vi "Get SMO PGSQL Log Paths.vi"(5 "getAll Cluster":variant, 7 "Default Paths":string, 8 "error in (no error)":errorcluster, 11 "FP-TC-Shared in":refnum<class "FP-TC-Shared.lvclass">) -> (0 "error out":errorcluster, 2 "Paths":string, 3 "FP-TC-Shared out":refnum<class "FP-TC-Shared.lvclass">)   [LabVIEW 2019, in "FP-TC-Shared.lvclass"]
uses:
  FP-TC-Shared.lvclass
  typedefs/Default PGSQL Paths.ctl
  FP-TC-Shared.lvclass/FP-TC-Shared.ctl
  <userlib>/LevyLab/Configuration/Configuration.lvclass/Configuration.ctl
  73a01e10-25b7-4c77-987b-687e2f0d43b2.vi
  <vilib>/Utility/Data Type/Get Type Information.vi
  <vilib>/Utility/Data Type/Get Numeric Information.vi
  <userlib>/_OpenG.lib/lvdata/lvdata.llb/Unwrap VVariant__ogtk.vi
  <userlib>/LevyLab/Instrument Framework/Instrument Types/Cryostat/Instrument.Cryostat.lvclass
  <userlib>/LevyLab/Configuration/Configuration.lvclass
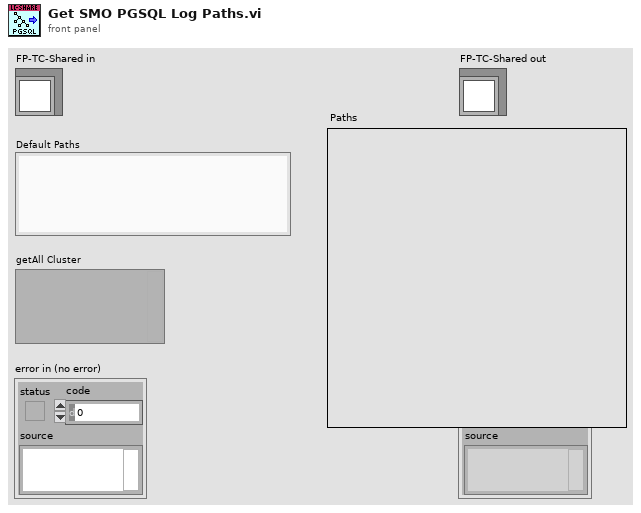
[diagram p1: front panel]
types:
  T1 = typedef "FP-TC-Shared.lvclass/Default PGSQL Paths.ctl" = cluster{"CF.TC":string, "CF.TC.Z":string, "CF.FP":string, "MNK.TC":string, "MNK.TC.Z":string, "MNK.FP":string}
  T2 = typedef "FP-TC-Shared.lvclass/LC Type--Enum.ctl" = enum16{"CF.TC", "CF.TC.Z", "CF.FP", "MNK.TC", "MNK.TC.Z", "MNK.FP"}
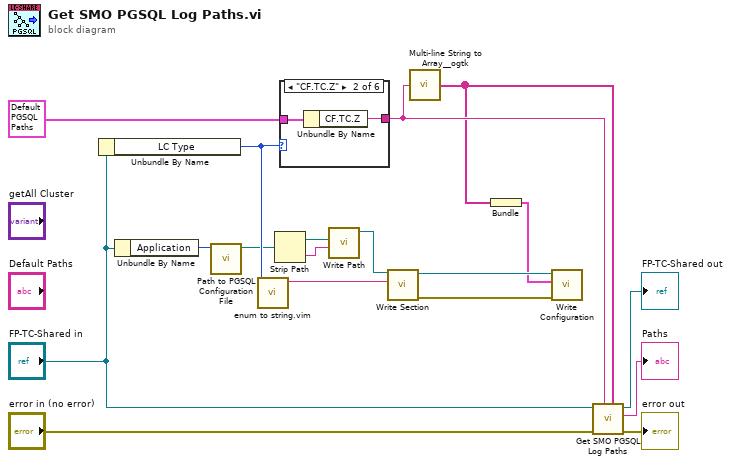
[diagram p0: block diagram]
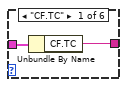
[diagram p2: hidden frame]
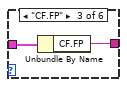
[diagram p3: hidden frame]
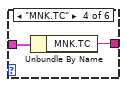
[diagram p4: hidden frame]
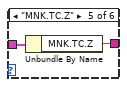
[diagram p5: hidden frame]
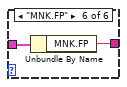
[diagram p6: hidden frame]
diagram:
  n1 = Unbundle By Name("FP-TC-Shared in") -> ("LC Type"=w12:T2)
  n2 = Unbundle By Name("FP-TC-Shared in") -> ("Application"=w6:enum16{"TC", "FP"})
  n3 = call "Path to PGSQL Configuration File.vi"("Application"=w6) -> ("appended path"=w2:path)  [unwired: 10 in]
  n4 = call "enum to string.vim"("enum in"=w12) -> ("string out"=w11:string)  [unwired: 9 in, 1 out]
  n5 = Strip Path(path=w2) -> (stripped path=w4:path, name=w5:string)
  n6 = case shown="\"CF.TC.Z\"" w12 {
    tunnel: T1 {"CF.TC"="llab_015:d001(Leiden CF900--CF_TC_R0(ohms))\nllab_015:d002(Leiden CF900--CF_TC_R1(ohms))\nllab_015:d003(Leiden CF900--CF_TC_R2(ohms))\nllab_015:d004(Leiden CF900--CF_TC_R3(ohms))\nllab_015:d005(Leiden CF900--CF_TC_R4(ohms))\nllab_015:d006(Leiden CF900--CF_TC_R5(ohms))\nllab_015:d007(Leiden CF900--CF_TC_R6(ohms))\nllab_015:d008(Leiden CF900--CF_TC_R7(ohms))\nllab_015:d009(Leiden CF900--CF_TC_T0(mK))\nllab_015:d010(Leiden CF900--CF_TC_T1(mK))\nllab_015:d011(Leiden CF900--CF_TC_T2(mK))\nllab_015:d012(Leiden CF900--CF_TC_T3(mK))\nllab_015:d013(Leiden CF900--CF_TC_T4(mK))\nllab_015:d014(Leiden CF900--CF_TC_T5(mK))\nllab_015:d015(Leiden CF900--CF_TC_T6(mK))\nllab_015:d016(Leiden CF900--CF_TC_T7(mK))\nllab_015:d017(Leiden CF900--CF_TC_I0(Amp))\nllab_015:d018(Leiden CF900--CF_TC_I1(Amp))\nllab_015:d019(Leiden CF900--CF_TC_I2(Amp))\nllab_015:d020(Leiden CF900--CF_TC_I3(Amp))\nllab_015:v000(Leiden CF900--CF_TC_description())\nllab_015:v001(Leiden CF900--CF_TC_calibration())", "CF.TC.Z"="llab_015:d021(Leiden CF900--CF_TC_Z_R0(ohms))\nllab_015:d022(Leiden CF900--CF_TC_Z_R1(ohms))\nllab_015:d023(Leiden CF900--CF_TC_Z_R2(ohms))\nllab_015:d024(Leiden CF900--CF_TC_Z_R3(ohms))\nllab_015:d025(Leiden CF900--CF_TC_Z_R4(ohms))\nllab_015:d026(Leiden CF900--CF_TC_Z_R5(ohms))\nllab_015:d027(Leiden CF900--CF_TC_Z_R6(ohms))\nllab_015:d028(Leiden CF900--CF_TC_Z_R7(ohms))\nllab_015:d029(Leiden CF900--CF_TC_Z_R8(ohms))\nllab_015:d030(Leiden CF900--CF_TC_Z_R9(ohms))\nllab_015:d031(Leiden CF900--CF_TC_Z_T0(mK))\nllab_015:d032(Leiden CF900--CF_TC_Z_T1(mK))\nllab_015:d033(Leiden CF900--CF_TC_Z_T2(mK))\nllab_015:d034(Leiden CF900--CF_TC_Z_T3(mK))\nllab_015:d035(Leiden CF900--CF_TC_Z_T4(mK))\nllab_015:d036(Leiden CF900--CF_TC_Z_T5(mK))\nllab_015:d037(Leiden CF900--CF_TC_Z_T6(mK))\nllab_015:d038(Leiden CF900--CF_TC_Z_T7(mK))\nllab_015:d039(Leiden CF900--CF_TC_Z_T8(mK))\nllab_015:d040(Leiden CF900--CF_TC_Z_T9(mK))\nllab_015:v002(Leiden CF900--CF_TC_Z_description())\nllab_015:v003(Leiden CF900--CF_TC_Z_calibration())", "CF.FP"="llab_011:d000(Leiden CF FP--CF_FP_P1(mbar))\nllab_011:d001(Leiden CF FP--CF_FP_P2(mbar))\nllab_011:d002(Leiden CF FP--CF_FP_P3(mbar))\nllab_011:d003(Leiden CF FP--CF_FP_P4(mbar))\nllab_011:d004(Leiden CF FP--CF_FP_P5(mbar))\nllab_011:d005(Leiden CF FP--CF_FP_P6(mbar))\nllab_011:d006(Leiden CF FP--CF_FP_P7(mbar))\nllab_011:d007(Leiden CF FP--CF_FP_Flow())\nllab_011:d008(Leiden CF FP--CF_FP_MG0(mbar))\nllab_011:d009(Leiden CF FP--CF_FP_MG1(mbar))\nllab_011:d010(Leiden CF FP--CF_FP_MG2(mbar))\nllab_011:d011(Leiden CF FP--CF_FP_MG3(mbar))\nllab_011:d012(Leiden CF FP--CF_FP_MG4(mbar))\nllab_011:d013(Leiden CF FP--CF_FP_MG5(mbar))\nllab_011:d014(Leiden CF FP--CF_FP_PT_on())\nllab_011:d015(Leiden CF FP--CF_FP_PT_W_in_T(K))\nllab_011:d016(Leiden CF FP--CF_FP_PT_W_out_T(K))\nllab_011:d017(Leiden CF FP--CF_FP_PT_He_T(K))\nllab_011:d018(Leiden CF FP--CF_FP_PT_oil_T(K))\nllab_011:d019(Leiden CF FP--CF_FP_PT_P_Low(bar))\nllab_011:d020(Leiden CF FP--CF_FP_PT_P_High(bar))\nllab_011:d021(Leiden CF FP--CF_FP_PT_current(A))\nllab_011:d022(Leiden CF FP--CF_FP_state0())\nllab_011:d023(Leiden CF FP--CF_FP_state1())\nllab_011:d024(Leiden CF FP--CF_FP_state2())\nllab_011:v000(Leiden CF FP--CF_FP_STATE())", "MNK.TC"="llab_024:d020(MNK_18T--MNK_TC_R0(ohms))\nllab_024:d039(MNK_18T--MNK_TC_R1(ohms))\nllab_024:d021(MNK_18T--MNK_TC_R2(ohms))\nllab_024:d022(MNK_18T--MNK_TC_R3(ohms))\nllab_024:d037(MNK_18T--MNK_TC_R4(ohms))\nllab_024:d023(MNK_18T--MNK_TC_R5(ohms))\nllab_024:d024(MNK_18T--MNK_TC_R6(ohms))\nllab_024:d025(MNK_18T--MNK_TC_R7(ohms))\nllab_024:d026(MNK_18T--MNK_TC_T0(mK))\nllab_024:d027(MNK_18T--MNK_TC_T1(mK))\nllab_024:d028(MNK_18T--MNK_TC_T2(mK))\nllab_024:d029(MNK_18T--MNK_TC_T3(mK))\nllab_024:d030(MNK_18T--MNK_TC_T4(mK))\nllab_024:d038(MNK_18T--MNK_TC_T5(mK))\nllab_024:d031(MNK_18T--MNK_TC_T6(mK))\nllab_024:d032(MNK_18T--MNK_TC_T7(mK))\nllab_024:d033(MNK_18T--MNK_TC_I0(Amp))\nllab_024:d034(MNK_18T--MNK_TC_I1(Amp))\nllab_024:d035(MNK_18T--MNK_TC_I2(Amp))\nllab_024:d036(MNK_18T--MNK_TC_I3(Amp))\nllab_024:v005(MNK_18T--MNK_TC_description())\nllab_024:v006(MNK_18T--MNK_TC_calibration())", "MNK.TC.Z"="llab_024:d040(MNK_18T--MNK_Cstill_Z(pF))\nllab_024:d041(MNK_18T--MNK_CMN-187_Z(H))\nllab_024:d042(MNK_18T--MNK_Cstill_T(mK))\nllab_024:d043(MNK_18T--MNK_CMN-187_T(mK))\nllab_024:v005(MNK_18T--MNK_TC_Z_description())\nllab_024:v006(MNK_18T--MNK_TC_Z_calibration())", "MNK.FP"="llab_016:d000(Leiden MNK Front Panel--MNK_FP_P1(mbar))\nllab_016:d001(Leiden MNK Front Panel--MNK_FP_P2(mbar))\nllab_016:d002(Leiden MNK Front Panel--MNK_FP_P3(mbar))\nllab_016:d003(Leiden MNK Front Panel--MNK_FP_P4(mbar))\nllab_016:d004(Leiden MNK Front Panel--MNK_FP_P5(mbar))\nllab_016:d005(Leiden MNK Front Panel--MNK_FP_P6(mbar))\nllab_016:d006(Leiden MNK Front Panel--MNK_FP_P7(mbar))\nllab_016:d013(Leiden MNK Front Panel--MNK_FP_Flow())\nllab_016:d007(Leiden MNK Front Panel--MNK_FP_MG0(mbar))\nllab_016:d008(Leiden MNK Front Panel--MNK_FP_MG1(mbar))\nllab_016:d009(Leiden MNK Front Panel--MNK_FP_MG2(mbar))\nllab_016:d010(Leiden MNK Front Panel--MNK_FP_MG3(mbar))\nllab_016:d011(Leiden MNK Front Panel--MNK_FP_MG4(mbar))\nllab_016:d012(Leiden MNK Front Panel--MNK_FP_MG5(mbar))\nllab_016:d014(Leiden MNK Front Panel--MNK_FP_state0())\nllab_016:d015(Leiden MNK Front Panel--MNK_FP_state1())\nllab_016:d016(Leiden MNK Front Panel--MNK_FP_state2())\nllab_016:v000(Leiden MNK Front Panel--MNK_FP_STATE())"} ("PGSQL Paths") -> [w20 w22 w24 w26 w28 w30]
    tunnel: [w19 w21 w23 w25 w27 w29] -> w13
    frame "CF.TC" {
      n7 = Unbundle By Name(w20) -> ("CF.TC"=w19:string)
    }
    frame "CF.TC.Z" {
      n8 = Unbundle By Name(w22) -> ("CF.TC.Z"=w21:string)
    }
    frame "CF.FP" {
      n9 = Unbundle By Name(w24) -> ("CF.FP"=w23:string)
    }
    frame "MNK.TC" {
      n10 = Unbundle By Name(w26) -> ("MNK.TC"=w25:string)
    }
    frame "MNK.TC.Z" {
      n11 = Unbundle By Name(w28) -> ("MNK.TC.Z"=w27:string)
    }
    frame "MNK.FP" {
      n12 = Unbundle By Name(w30) -> ("MNK.FP"=w29:string)
    }
  }
  n13 = call <userlib>:"Write Path.vi"("Filename [Configuration.ini]"=w5, "Path"=w4) -> ("Configuration out"=w1:refnum<class "Configuration.lvclass">)  [unwired: 8 in, 1 out]
  n14 = call <userlib>:"Write Section.vi"("Section"=w11, "Configuration in"=w1) -> ("error out"=w10:errorcluster, "Configuration out"=w9:refnum<class "Configuration.lvclass">)  [unwired: 8 in]
  n15 = call <userlib>:"Multi-line String to Array__ogtk.vi"("string"=w13) -> ("lines"=w8:string[])
  n16 = Bundle("lines"=w8) -> (w7:cluster{"lines":string[]})  [unwired: 1 in]
  n17 = call <userlib>:"Write Configuration.vi"("error in (no error)"=w10, "Variant"=w7, "Configuration in"=w9) -> ()  [unwired: 7 in, 2 out]
  n18 = call-parent "Get SMO PGSQL Log Paths.vi"("getAll Cluster"=w8, "Default Paths"=w13, "error in (no error)"="error in (no error)", "Instrument in"="FP-TC-Shared in") -> ("error out"=→"error out":errorcluster, "Paths"=→"Paths":string, "Instrument out"=→"FP-TC-Shared out":refnum<class "FP-TC-Shared.lvclass">)  [unwired: 5 in]
